vi "Select Save Location.vi"(8 "error in (no error)":errorcluster, 10 "Current Save Location":path) -> (0 "error out":errorcluster, 2 "New Save Location":path)   [LabVIEW 2018]
panel:
  in  "Continue":bool
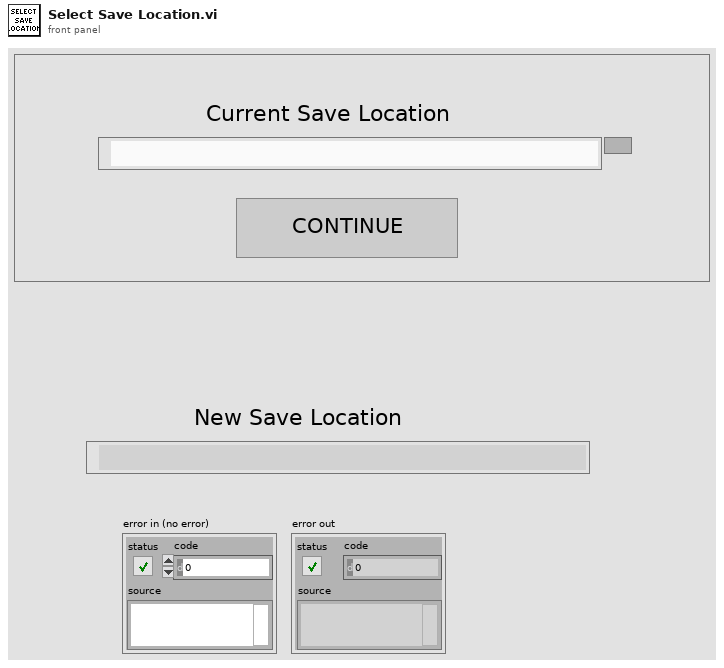
[diagram p1: front panel]
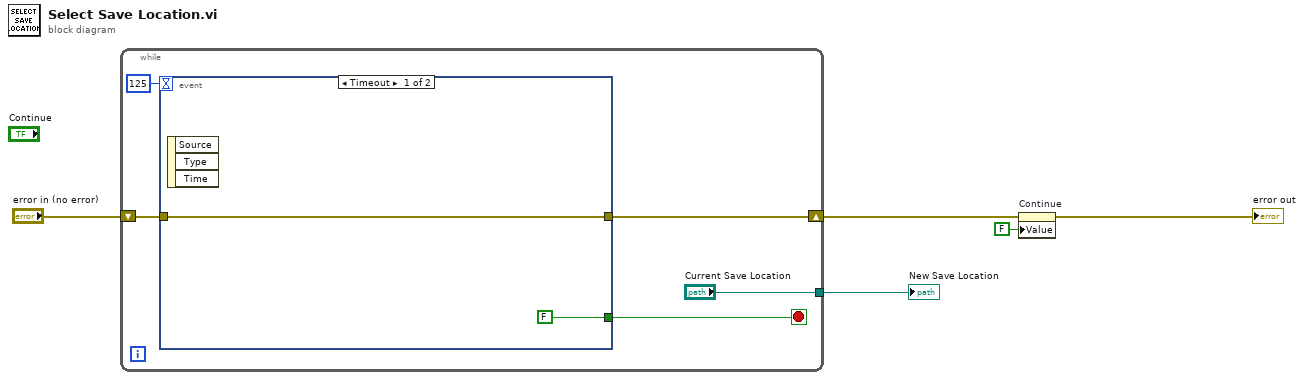
[diagram p0: block diagram]
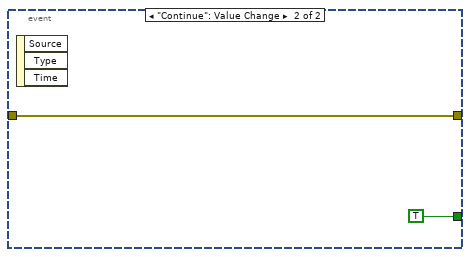
[diagram p2: hidden frame]
diagram:
  n1 = while {
    shift-right: [w7] -> w3
    shift-left: "error in (no error)" -> [w8]
    tunnel: ["Current Save Location"] -> w4
    stop <- w9 stop-if-true
    n2 = event shown="[0] Timeout" {
      selector: _ -> [_ _]
      dyn-events: _ -> [_ _]
      timeout: 125 -> [_ _]
      tunnel: [FALSE TRUE] -> w9
      tunnel: w8 -> [w11 w13]
      tunnel: [w11 w13] -> w7
      event Timeout {
        n3 = event-data() -> ()  [unwired: 1 in, 3 out]
      }
      event "Continue": Value Change {
        n4 = event-data() -> ()  [unwired: 1 in, 3 out]
      }
    }
  }
  "New Save Location" <- w4
  n5 = property on="Continue" class="Bool (strict)"(error in=w3, "Value"=FALSE ("Continue")) -> (error out=→"error out":errorcluster)  [unwired: 1 in, 1 out]
